vi "HandleExit.vi"(8 "error in (no error)":errorcluster, 9 "VI Refnum":refnum<vi>, 10 "StopArgument":variant, 11 "ModuleAdmin":refnum<class "ModuleAdmin.lvclass">) -> (0 "error out":errorcluster, 1 "Exit via Stop Module Req?":bool, 2 "WaitForStop?":bool)   [LabVIEW 2014, in "SyncModule.lvlib"]
uses:
  SyncModule.lvlib
  <userlib>/NIST/ModuleAdminLib/ModuleAdmin/ModuleAdmin.lvclass
  PublicAPI/Arguments/Requests/clStopArgument.ctl
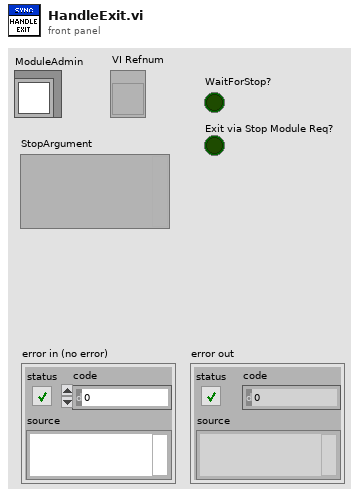
[diagram p1: front panel]
types:
  T1 = typedef "SyncModule.lvlib/clStopArgument.ctl" = cluster{"Exit via Stop Module Req?":bool, "Wait for Module to stop?":bool, "ModuleAdmin":refnum<class "ModuleAdmin.lvclass">}
  T2 = enum32{"Invalid", "Standard", "Closed", "Hidden", "Minimized", "Maximized"}
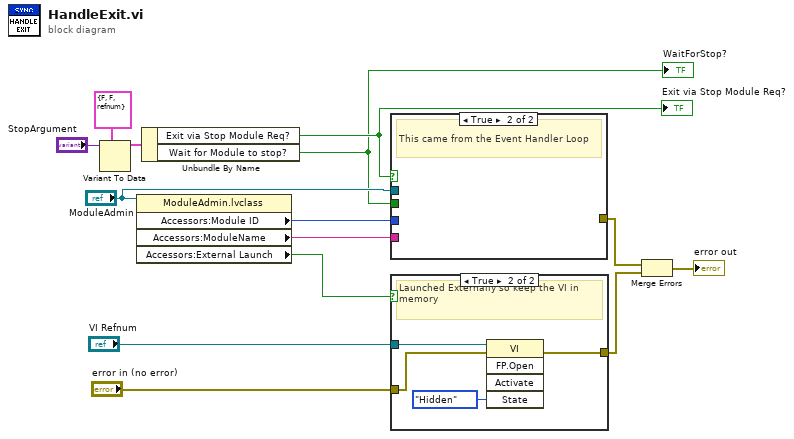
[diagram p0: block diagram]
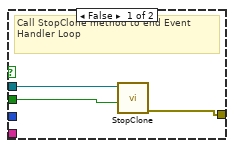
[diagram p3: hidden frame]
diagram:
  n1 = Variant To Data(type=T1 {"Exit via Stop Module Req?"=FALSE, "Wait for Module to stop?"=FALSE, "ModuleAdmin"=refnum} ("Stop Argument"), Variant="StopArgument") -> (data=w8:T1)  [unwired: 1 in, 1 out]
  n2 = property class="ModuleAdmin.lvclass"(reference="ModuleAdmin") -> ("Accessors:Module ID"=w4:i32, "Accessors:ModuleName"=w5:string, "Accessors:External Launch"=w6:bool)  [unwired: 1 in, 2 out]
  n3 = Unbundle By Name(w8) -> ("Exit via Stop Module Req?"=w3:bool, "Wait for Module to stop?"=w1:bool)
  "WaitForStop?" <- w1
  "Exit via Stop Module Req?" <- w3
  n4 = case shown="True" w3 {
    tunnel: w4 -> [_ _]
    tunnel: [w17 _] -> w12
    tunnel: w5 -> [_ _]
    tunnel: w1 -> [w16 _]
    tunnel: "ModuleAdmin" -> [w15 _]
    frame False {
      # "Call StopClone method to end Event Handler Loop"
      n5 = call "StopClone.vi"("Wait for Module to stop?"=w16, "ModuleAdmin"=w15) -> ("error out"=w17:errorcluster)  [unwired: 9 in]
    }
    frame True {
      # "This came from the Event Handler Loop"
    }
  }
  n6 = case shown="True" w6 {
    tunnel: "VI Refnum" -> [_ w22]
    tunnel: [w18 w20] -> w11
    tunnel: "error in (no error)" -> [w18 w19]
    frame False {
    }
    frame True {
      # "Launched Externally so keep the VI in memory"
      n7 = invoke class="VI" method="FP.Open"(reference=w22, error in=w19, "State"=T2."Hidden") -> (error out=w20:errorcluster)  [unwired: 2 in, 4 out]
    }
  }
  n8 = Merge Errors(w12, w11) -> (→"error out":errorcluster)
